vi "Read Measurement (Third Order Intercept IP3).vi"(0 "VISA resource name":refnum<visa-resource-name>, 11 "error in (no error)":errorcluster) -> (4 "VISA resource name out":refnum<visa-resource-name>, 6 "TOI Worst Value":dbl format="%.3f", 15 "error out":errorcluster)   [LabVIEW 2020, in "Anritsu Signal Analyzer Series.lvlib"]
doc: "Reads TOI IP3 and displays the worst value of TOI ."
uses:
  Anritsu Signal Analyzer Series.lvlib
panel:
  # "dB"
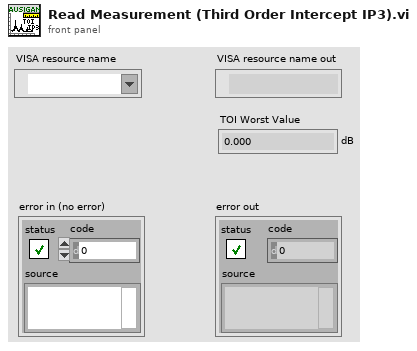
[diagram p1: front panel]
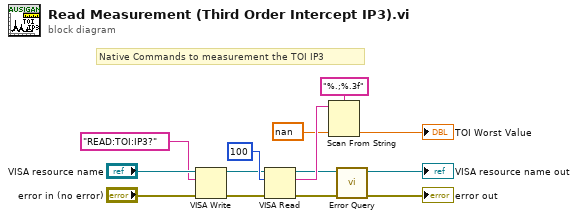
[diagram p0: block diagram]
diagram:
  # "Native Commands to measurement the TOI IP3"
  n1 = VISA Write(VISA resource name="VISA resource name", write buffer="READ:TOI:IP3?" ("_Command"), error in (no error)="error in (no error)") -> (VISA resource name out=w6:refnum<visa-resource-name>, error out=w7:errorcluster)  [unwired: 1 out]
  n2 = VISA Read(VISA resource name=w6, byte count=u32 100 ("byte count (0)"), error in (no error)=w7) -> (VISA resource name out=w2:refnum<visa-resource-name>, read buffer=w5:string, error out=w3:errorcluster)  [unwired: 1 out]
  n3 = Scan From String(format string="%.;%.3f" ("Format String"), input string=w5, default 1=nan ("_Default")) -> (output 1=→"TOI Worst Value":dbl)  [unwired: 2 in, 3 out]
  n4 = call "Error Query.vi"("error in (no error)"=w3, "VISA resource name"=w2) -> ("error out"=→"error out":errorcluster, "VISA resource name out"=→"VISA resource name out":refnum<visa-resource-name>)  [unwired: 6 in, 2 out]
